vi "UniPend - Linearizer.vi"(3 "Up-Up":bool) -> (5 "State-Space Model":T1 {"Transport Delay" format="%.2f"; "D" format="%#.2g"; "C" format="%#.2g"; "B" format="%#.2g"; "A" format="%#.2g"; "properties"."Sampling Time" format="%#.6p"; "properties"."Output Delays" format="%.4f"; "properties"."Input Delays" format="%.4f"})   [LabVIEW 2012]
uses:
  <vilib>/addons/Control Design/_Model Construction/Model Typedefs.llb/CD State Space Model (MIMO).ctl
  <vilib>/addons/Control Design/_Model Construction/Model Typedefs.llb/CD General Elements.ctl
  <vilib>/Simulation/Model Trim and Linearize/SIM Query Subsystem.llb/SIM Query Subsystem (Reference).vi
  <vilib>/Simulation/Model Trim and Linearize/SIM Linearize.llb/SIM Linearize (Reference).vi
  <vilib>/addons/Control Design/_Model Construction/Model Information.llb/Model Information SubVIs/cd_Get Names From SS Model.vi
  <vilib>/addons/Control Design/_Model Reduction/Model Reduction.llb/Model Reduction SubVIs/cd_Select I-O-S from SS Model.vi
  <vilib>/addons/Control Design/_Model Reduction/NI_CD_Model Reduction.lvlib
  <vilib>/addons/Control Design/_Model Construction/NI_LinSys_Model Information.lvlib
  <vilib>/addons/Control Design/_Model Construction/NI_LinSys_Model Typedefs.lvlib
panel:
  out "States Reorder":i32[](array[numeric])
  out "State Names":string[](array[string])
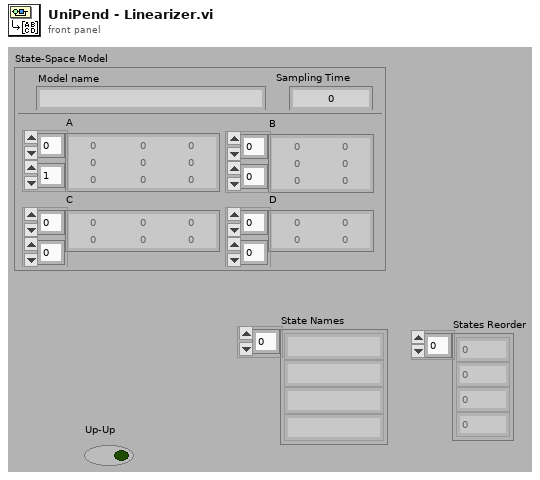
[diagram p1: front panel]
types:
  T1 = typedef "NI_LinSys_Model Typedefs.lvlib/CD State Space Model (MIMO).ctl" = cluster{"properties":T2, "A":dbl[][], "B":dbl[][], "C":dbl[][], "D":dbl[][], "StateNames":string[], "Transport Delay":dbl[][]}
  T2 = typedef "NI_LinSys_Model Typedefs.lvlib/CD General Elements.ctl" = cluster{"Model name":string, "Input names":string[], "Output names":string[], "Input Delays":dbl[], "Output Delays":dbl[], "Sampling Time":dbl, "Notes":string}
  T3 = typedef "SIM Trim or Lin Param.ctl" = cluster{"Name":string, "Value":dbl[], "Static Input?":bool, "Vector?":bool, "Fixed Size?":bool, "Fixed Value?":bool}
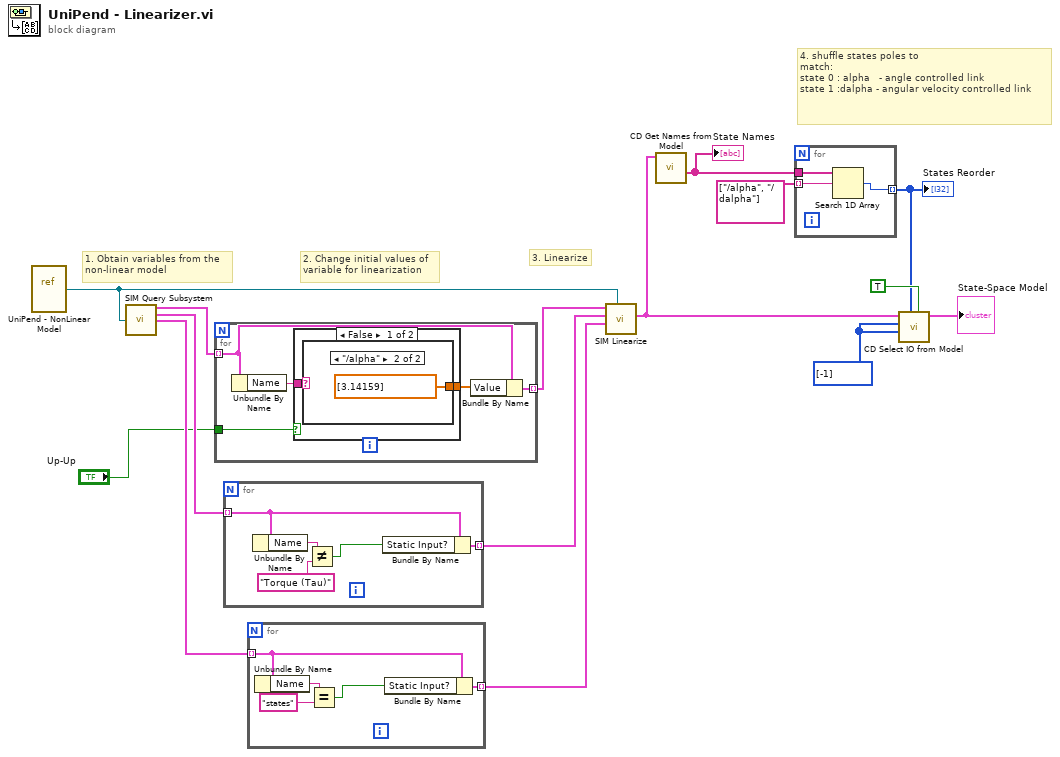
[diagram p0: block diagram]
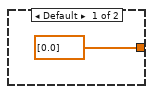
[diagram p2: hidden frame]
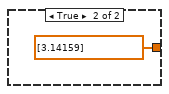
[diagram p3: hidden frame]
diagram:
  w7 = i32[] [-1] ("Inputs")
  # "4. shuffle states poles to\nmatch:\nstate 0 : alpha   - angle controlled link\nstate 1 :dalpha - angular velocity controlled link"
  # "3. Linearize"
  # "2. Change initial values of\nvariable for linearization"
  # "1. Obtain variables from the\nnon-linear model"
  n1 = vi-ref "UniPend - NonLinear Model.vi"() -> (w15:refnum<vi>)
  n2 = call-poly <vilib>:"SIM Query Subsystem.vi"("Reference"=w15) -> ("States"=w10:T3[], "Inputs"=w14:T3[], "Outputs"=w12:T3[])  [unwired: 12 out]
  n3 = for {
    tunnel: w10 -> [w19] mode=indexing
    tunnel: [w18] -> w9 mode=indexing
    tunnel: "Up-Up" -> [w16]
    n4 = Unbundle By Name(w19) -> ("Name"=w20:string)
    n5 = case shown="False" w16 {
      tunnel: w20 -> [w22 _]
      tunnel: [w21 dbl[] [3.14159] ("Value")] -> w17
      frame False {
        n6 = case shown="\"/alpha\"" w22 {
          tunnel: [dbl[] [0.0] ("Value") dbl[] [3.14159] ("Value")] -> w21
          frame Default {
          }
          frame "/alpha" {
          }
        }
      }
      frame True {
      }
    }
    n7 = Bundle By Name(cluster=w19, "Value"=w17) -> (w18:T3)
  }
  n8 = for {
    tunnel: w14 -> [w29] mode=indexing
    tunnel: [w30] -> w13 mode=indexing
    n9 = Unbundle By Name(w29) -> ("Name"=w28:string)
    n10 = Not Equal?(x=w28, y="Torque (Tau)") -> (x != y?=w26:bool)
    n11 = Bundle By Name(cluster=w29, "Static Input?"=w26) -> (w30:T3)
  }
  n12 = for {
    tunnel: w12 -> [w34] mode=indexing
    tunnel: [w35] -> w11 mode=indexing
    n13 = Unbundle By Name(w34) -> ("Name"=w33:string)
    n14 = Equal?(x=w33, y="states") -> (x = y?=w31:bool)
    n15 = Bundle By Name(cluster=w34, "Static Input?"=w31) -> (w35:T3)
  }
  n16 = call-poly <vilib>:"SIM Linearize.vi"("Reference"=w15, "Outputs"=w11, "Inputs"=w13, "States"=w9) -> ("State-Space Model"=w4:T1)  [unwired: 1 in, 6 out]
  n17 = call-poly <vilib>:"CD Get Names from Model.vi"("State-Space Model"=w4) -> ("State Names"=w2:string[])  [unwired: 5 in, 5 out]
  "State Names" <- w2
  n18 = for {
    tunnel: string[] ["/alpha", "/dalpha"] ("State Names") -> [w37] mode=indexing
    tunnel: w2 -> [w38]
    tunnel: [w36] -> w1 mode=indexing
    n19 = Search 1D Array(1D array=w38, element=w37) -> (index of element=w36:i32)  [unwired: 1 in]
  }
  "States Reorder" <- w1
  n20 = call-poly <vilib>:"CD Select IO from Model.vi"("State-Space Model"=w4, "Inputs"=w7, "Outputs"=w7, "States"=w1, "Allow Reorder"=TRUE) -> ("Selected Model"=→"State-Space Model":T1)  [unwired: 1 in, 4 out]
